vi "Create New Report.vi"(8 "error in (no error)":errorcluster, 9 "Report Path":path, 11 "OnTheFlyReport in":refnum<class "OnTheFlyReport.lvclass">) -> (0 "error out":errorcluster, 3 "OnTheFlyReport out":refnum<class "OnTheFlyReport.lvclass">)   [LabVIEW 2015, in "OnTheFlyReport.lvclass"]
uses:
  OnTheFlyReport.lvclass
  OnTheFlyReport.lvclass/OnTheFlyReport.ctl
  Report Formatters/Base Class/Execution/Formatter.lvclass
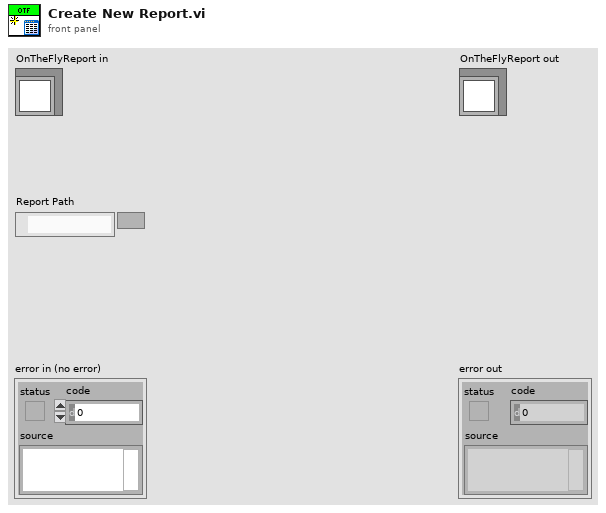
[diagram p1: front panel]
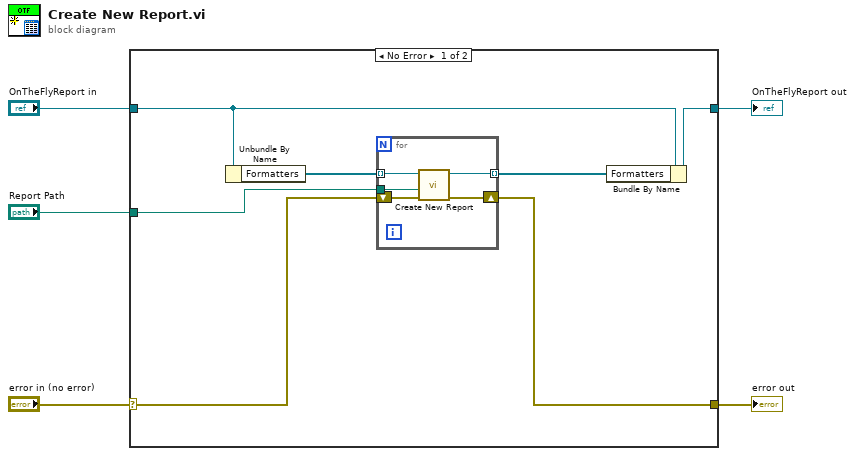
[diagram p0: block diagram]
diagram:
  n1 = case shown="No Error" "error in (no error)" {
    selector: "error in (no error)" -> [w10 w19]
    tunnel: [w9 w19] -> w4
    tunnel: [w7 w18] -> w3
    tunnel: "OnTheFlyReport in" -> [w12 w18]
    tunnel: "Report Path" -> [w8 _]
    frame No Error {
      n2 = Unbundle By Name(w12) -> ("Formatters"=w11:refnum<class "Formatter.lvclass">[])
      n3 = for {
        tunnel: w11 -> [w17] mode=indexing
        shift-right: [w15] -> w9
        shift-left: w10 -> [w16]
        tunnel: w8 -> [w14]
        tunnel: [w13] -> w6 mode=indexing
        n4 = call-dynamic "Create New Report.vi"("error in (no error)"=w16, "Report Path"=w14, "Formatter in"=w17) -> ("error out"=w15:errorcluster, "Formatter out"=w13:refnum<class "Formatter.lvclass">)  [unwired: 7 in]
      }
      n5 = Bundle By Name(cluster=w12, "Formatters"=w6) -> (w7:refnum<class "OnTheFlyReport.lvclass">)
    }
    frame Error {
    }
  }
  "error out" <- w4
  "OnTheFlyReport out" <- w3
